vi "PWM Output DAQ Engine.vi"(8 "error in":errorcluster, 10 "DAQ Engine":refnum<notifier>, 11 "Sequence Context In":refnum<k7>) -> (0 "error out":errorcluster)   [LabVIEW 2023, in "LTT_TeststandSteptypes.lvlib"]
uses:
  LTT_TeststandSteptypes.lvlib
  HardwareAbstractionLayer_LVOOP/Main/Class Ref.ctl
  HardwareAbstractionLayer_LVOOP/DMM/DMM.lvclass
  HardwareAbstractionLayer_LVOOP/Function Generator/Function Generator.lvclass
  HardwareAbstractionLayer_LVOOP/Oscilloscope/Oscilloscope.lvclass
  HardwareAbstractionLayer_LVOOP/PowerSupply/PowerSupply.lvclass
  HardwareAbstractionLayer_LVOOP/Teststand/Teststand.lvclass
  HardwareAbstractionLayer_LVOOP/Analog Output/AO/AO.lvclass
  HardwareAbstractionLayer_LVOOP/Analog Input/AI/AI.lvclass
  HardwareAbstractionLayer_LVOOP/Database/Database.lvclass
  HardwareAbstractionLayer_LVOOP/Digital Output/DO_class/DO.lvclass
  HardwareAbstractionLayer_LVOOP/Digital Input/DI_class/DI.lvclass
  HardwareAbstractionLayer_LVOOP/PWM Output/PWM Output_class/PWM Output.lvclass
  HardwareAbstractionLayer_LVOOP/PWM Input/PWM Input_class/PWM Input.lvclass
  HardwareAbstractionLayer_LVOOP/NI Switch/NISwitch_class/NISwitch.lvclass
  HardwareAbstractionLayer_LVOOP/Modbus/Modbus_class/Modbus.lvclass
  HardwareAbstractionLayer_LVOOP/CAN/CAN Lib/CAN_class/CAN.lvclass
  HardwareAbstractionLayer_LVOOP/PWM Output/NI PWM Output_class/NI PWM Output.lvclass
  D:/eDCU LTT/VT LTT Project/Source Code/HardwareAbstractionLayer_LVOOP/PWM Output/PWM Output_class/PWM Output.lvclass
  HardwareAbstractionLayer_LVOOP/Main/Class Options.ctl
  PWM Output/Control/PWM Output Data.ctl
  <vilib>/Utility/error.llb/DialogType.ctl
  HardwareAbstractionLayer_LVOOP/Main/Main.lvclass
  D:/eDCU LTT/VT LTT Project/Source Code/HardwareAbstractionLayer_LVOOP/PWM Output/NI PWM Output_class/NI PWM Output.lvclass
panel:
  in  "stop":bool
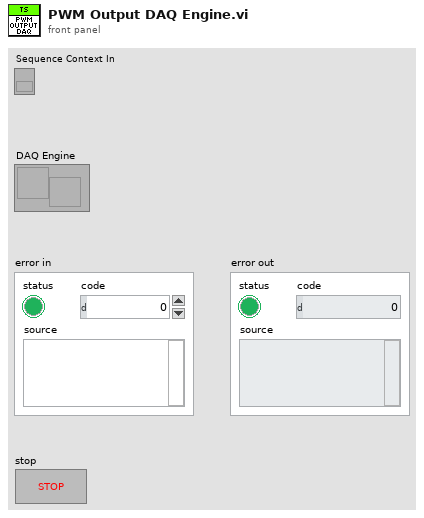
[diagram p1: front panel]
types:
  T1 = typedef "HardwareAbstractionLayer_LVOOP.lvlib/Main.lvclass/Class Ref.ctl" = cluster{"DMM":refnum<class "DMM.lvclass">, "Function Generator":refnum<class "Function Generator.lvclass">, "Oscilloscope":refnum<class "Oscilloscope.lvclass">, "PowerSupply":refnum<class "PowerSupply.lvclass">, "Teststand":refnum<class "Teststand.lvclass">, "AO":refnum<class "AO.lvclass">, "AI":refnum<class "AI.lvclass">, "Database":refnum<class "Database.lvclass">, "AO Waveform Generation":refnum<class "AO.lvclass">, "DO":refnum<class "DO.lvclass">, "DI":refnum<class "DI.lvclass">, "PWM Output":refnum<class "PWM Output.lvclass">, "PWM Input":refnum<class "PWM Input.lvclass">, "RelayOutput":refnum<class "NISwitch.lvclass">, "Modbus":refnum<class "Modbus.lvclass">, "CAN":refnum<class "CAN.lvclass">}
  T2 = typedef "HardwareAbstractionLayer_LVOOP.lvlib/Main.lvclass/Class Options.ctl" = enum16{"Init All Class", "Read All Class", "Write AI Class", "Write AO Class", "Write AO Waveform Generation", "Write DI Class", "Write DO Class", "Write PWM Input Class", "Write PWM Output Class", "Exit"}
  T3 = typedef "LTT_TeststandSteptypes.lvlib/PWM Output Data.ctl" = cluster{"Frequency":dbl, "Duty Cycle":dbl, "PWM Action":enum16{"PWM Start", "PWM Stop"}}
  T4 = typedef "DialogType.ctl" = u16
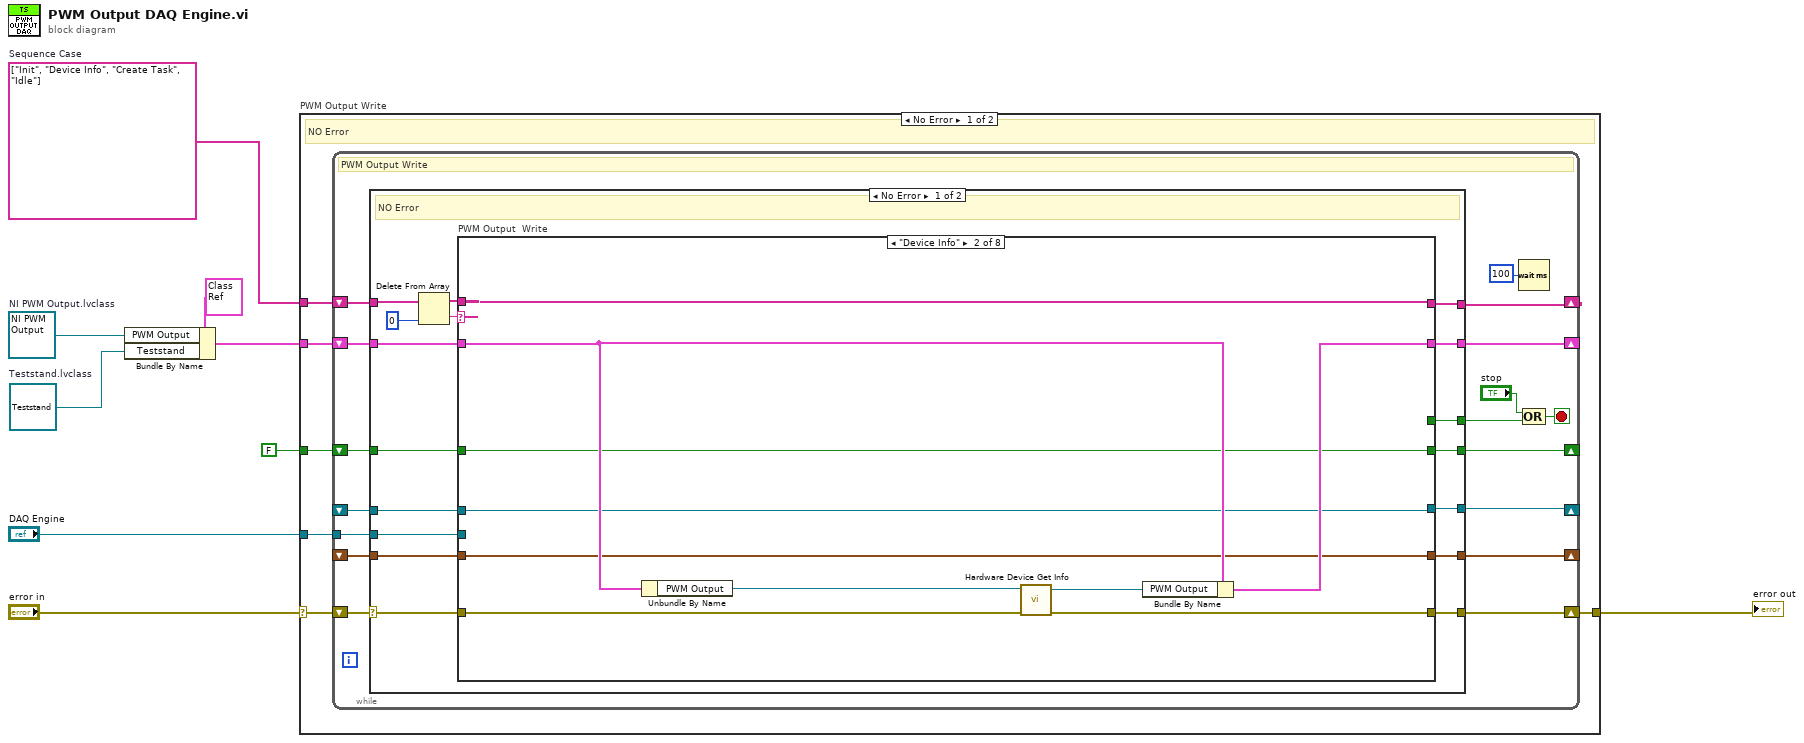
[diagram p0: block diagram]
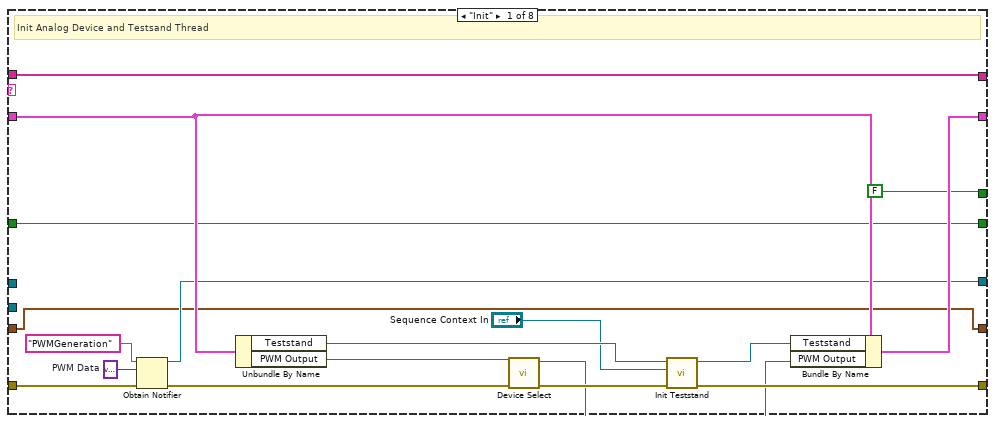
[diagram p2: hidden frame]
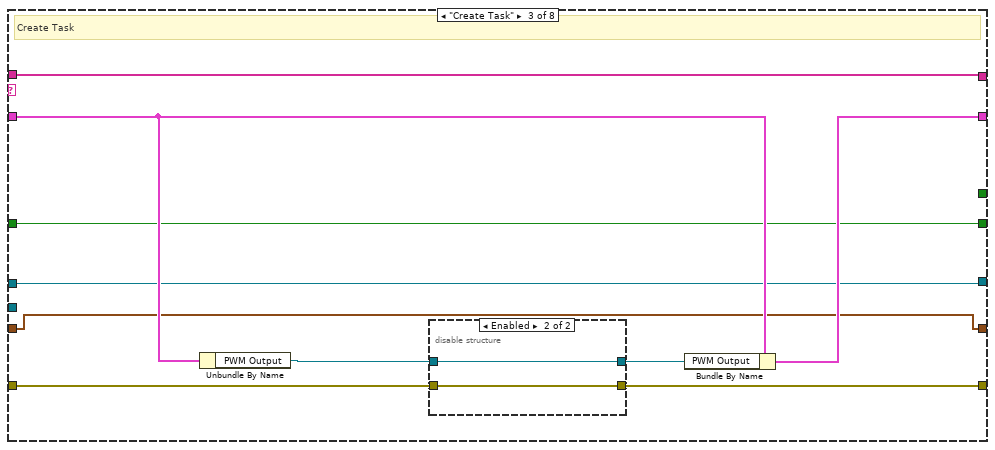
[diagram p3: hidden frame]
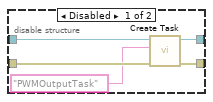
[diagram p4: hidden frame]
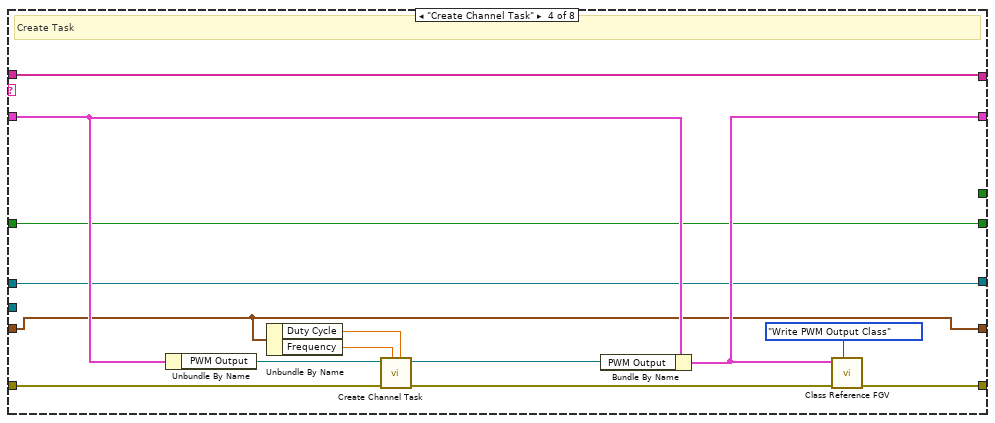
[diagram p5: hidden frame]
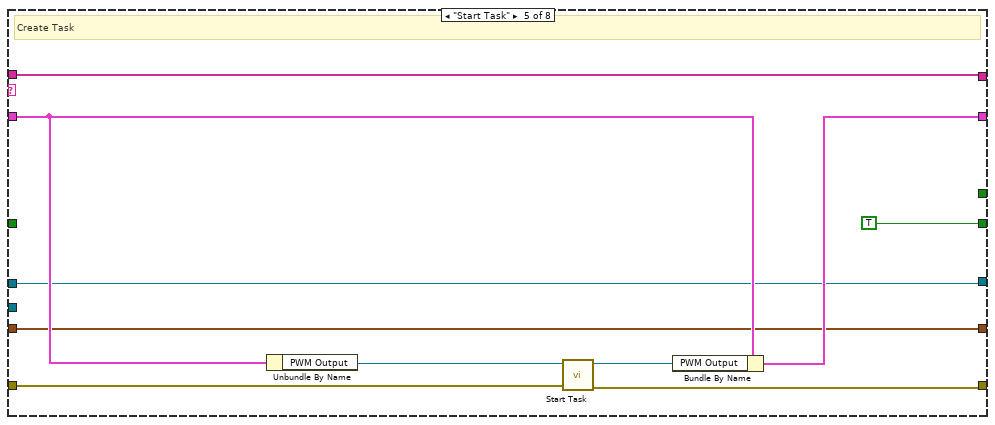
[diagram p6: hidden frame]
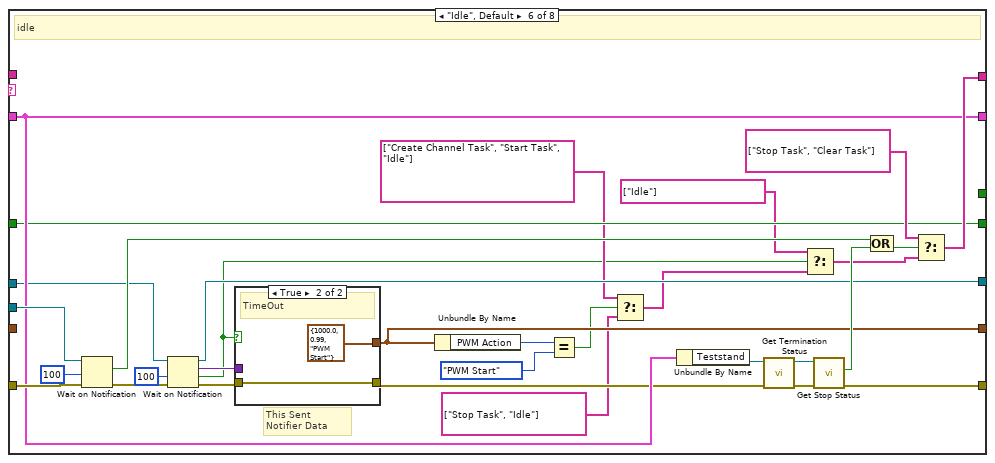
[diagram p7: hidden frame]
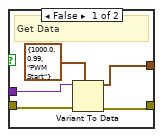
[diagram p8: hidden frame]
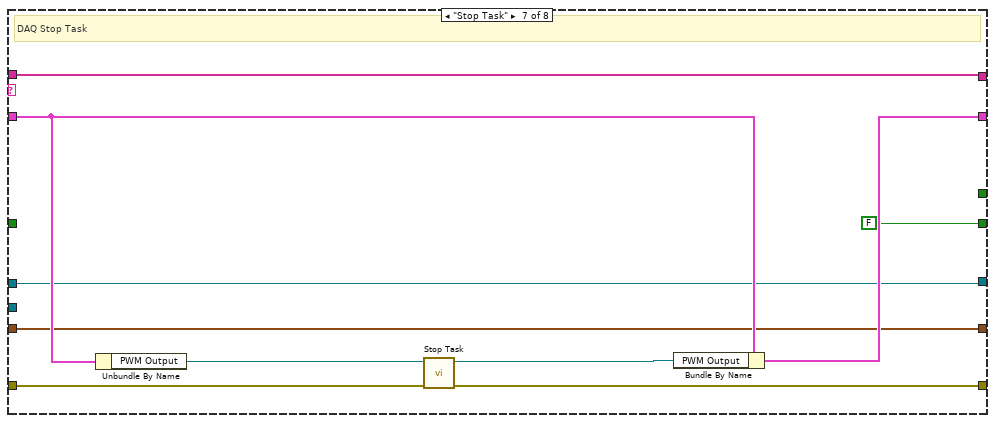
[diagram p9: hidden frame]
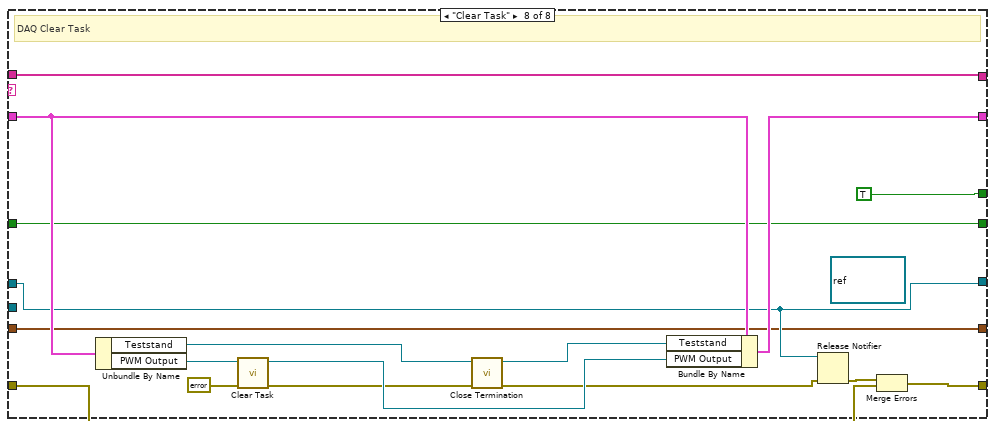
[diagram p10: hidden frame]
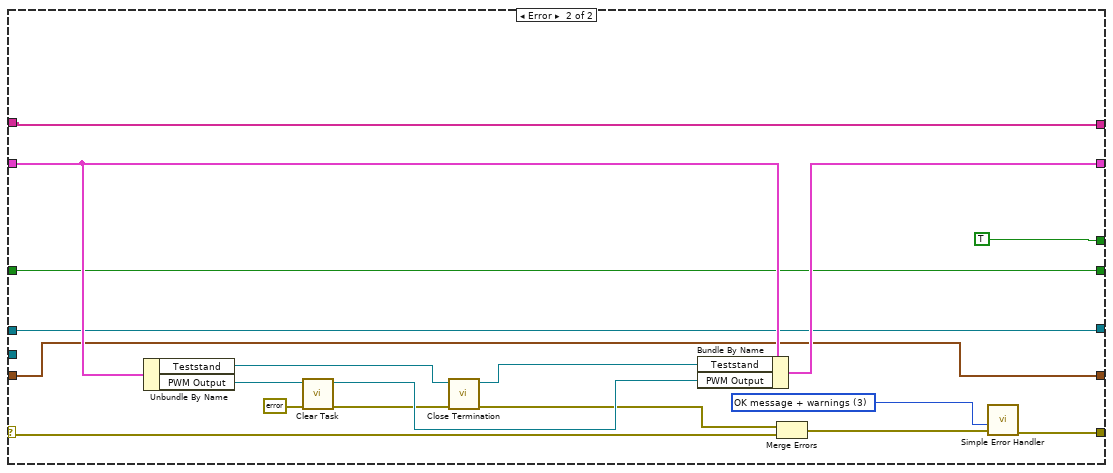
[diagram p11: hidden frame]
diagram:
  w4 = refnum<class "Teststand.lvclass"> refnum  # Teststand.lvclass
  w5 = refnum<class "NI PWM Output.lvclass"> refnum  # NI PWM Output.lvclass
  w7 = string[] ["Init", "Device Info", "Create Task", "Idle"]  # Sequence Case
  n1 = Bundle By Name(cluster=T1 {"DMM"=refnum, "Function Generator"=refnum, "Oscilloscope"=refnum, "PowerSupply"=refnum, "Teststand"=refnum, "AO"=refnum, "AI"=refnum, "Database"=refnum, "AO Waveform Generation"=refnum, "DO"=refnum, "DI"=refnum, "PWM Output"=refnum, "PWM Input"=refnum, "RelayOutput"=refnum, "Modbus"=refnum, "CAN"=refnum} ("Class Cluster"), "PWM Output"=w5, "Teststand"=w4) -> (w8:T1)
  n2 = case "PWM Output Write" shown="No Error" "error in" {
    selector: "error in" -> [w15 w202]
    tunnel: [w14 w202] -> w1
    tunnel: w8 -> [w13 _]
    tunnel: w7 -> [w12 _]
    tunnel: "DAQ Engine" -> [w11 _]
    tunnel: FALSE -> [w10 _]
    frame No Error {
      # "NO Error"
      n3 = while {
        shift-right: [w31] -> w14
        shift-left: w15 -> [w32]
        shift-right: [w29] -> _
        shift-left: w13 -> [w30]
        shift-right: [w27] -> _
        shift-left: w12 -> [w28]
        tunnel: w11 -> [w22]
        shift-right: [w21] -> _
        shift-left: _ -> [w20]
        shift-right: [w18] -> _
        shift-left: w10 -> [w19]
        shift-right: [w17] -> _
        shift-left: _ -> [w16]
        stop <- w24 stop-if-true
        # "PWM Output Write"
        n4 = case shown="No Error" w32 {
          selector: w32 -> [w49 w193]
          tunnel: [w48 w187] -> w31
          tunnel: w30 -> [w44 w191]
          tunnel: [w43 w192] -> w29
          tunnel: w28 -> [w47 w190]
          tunnel: [w41 w190] -> w27
          tunnel: [w40 TRUE] -> w23
          tunnel: w22 -> [w39 _]
          tunnel: [w38 w189] -> w21
          tunnel: w20 -> [w37 w189]
          tunnel: w19 -> [w36 w185]
          tunnel: [w35 w185] -> w18
          tunnel: [w34 w184] -> w17
          tunnel: w16 -> [w33 w184]
          frame No Error {
            # "NO Error"
            n5 = Delete From Array(array=w47, index=0) -> (deleted portion=w46:string, array with subset deleted=w42:string[])  [unwired: 1 in]
            n6 = case "PWM Output  Write" shown="\"Device Info\"" w46 {
              tunnel: w49 -> [w55 w74 w84 w106 w115 w149 w163 w172]
              tunnel: [w59 w73 w83 w102 w113 w142 w158 w173] -> w48
              tunnel: w44 -> [w66 w76 w86 w107 w117 w140 w165 w182]
              tunnel: [w65 w75 w85 w100 w116 w140 w164 w181] -> w43
              tunnel: w42 -> [w67 w77 w87 w108 w118 _ w166 w183]
              tunnel: [w67 w77 w87 w108 w118 w147 w166 w183] -> w41
              tunnel: [FALSE _ _ _ _ _ _ TRUE] -> w40
              tunnel: w39 -> [_ _ _ _ _ w145 _ _]
              tunnel: [w53 w70 w80 w99 w111 w136 w161 w171] -> w38
              tunnel: w37 -> [_ w70 w80 w99 w111 w130 w161 w171]
              tunnel: w36 -> [w52 w69 w79 w98 _ w134 _ w168]
              tunnel: [w52 w69 w79 w98 TRUE w134 FALSE w168] -> w35
              tunnel: [w50 w68 w78 w97 w109 w129 w157 w167] -> w34
              tunnel: w33 -> [w50 w68 w78 w97 w109 _ w157 w167]
              frame "Init" {
                w51 = variant  # PWM Data
                # "Init Analog Device and Testsand Thread"
                n7 = Obtain Notifier(name (unnamed)="PWMGeneration", notification data type=w51, error in (no error)=w55) -> (notifier out=w53:refnum<notifier>, error out=w54:errorcluster)  [unwired: 1 in, 1 out]
                n8 = Unbundle By Name(w66) -> ("Teststand"=w62:refnum<class "Teststand.lvclass">, "PWM Output"=w63:refnum<class "PWM Output.lvclass">)
                n9 = call-dynamic "Device Select.vi"("error in (no error)"=w54, "PWM Output in"=w63) -> ("error out"=w60:errorcluster, "PWM Output out"=w57:refnum<class "PWM Output.lvclass">)  [unwired: 8 in]
                n10 = call-dynamic "Init Teststand.vi"("error in (no error)"=w60, "Sequence Context In"="Sequence Context In", "Teststand in"=w62) -> ("error out"=w59:errorcluster, "Teststand out"=w58:refnum<class "Teststand.lvclass">)  [unwired: 7 in]
                n11 = Bundle By Name(cluster=w66, "Teststand"=w58, "PWM Output"=w57) -> (w65:T1)
              }
              frame "Device Info" {
                n12 = Unbundle By Name(w76) -> ("PWM Output"=w71:refnum<class "PWM Output.lvclass">)
                n13 = call-dynamic "Hardware Device Get Info.vi"("error in (no error)"=w74, "PWM Output in"=w71) -> ("error out"=w73:errorcluster, "PWM Output out"=w72:refnum<class "PWM Output.lvclass">)  [unwired: 8 in]
                n14 = Bundle By Name(cluster=w76, "PWM Output"=w72) -> (w75:T1)
              }
              frame "Create Task" {
                # "Create Task"
                n15 = Unbundle By Name(w86) -> ("PWM Output"=w81:refnum<class "PWM Output.lvclass">)
                n16 = disable-structure shown="Enabled" {
                  disable-tunnel: w84 -> [w92 w93]
                  disable-tunnel: [w91 w93] -> w83
                  disable-tunnel: [w90 w94] -> w82
                  disable-tunnel: w81 -> [w89 w94]
                  frame Disabled {
                    n17 = call-dynamic "Create Task.vi"("error in (no error)"=w92, "Task name"="PWMOutputTask", "PWM Output in"=w89) -> ("error out"=w91:errorcluster, "PWM Output out"=w90:refnum<class "PWM Output.lvclass">)  [unwired: 7 in]
                  }
                  frame Enabled {
                  }
                }
                n18 = Bundle By Name(cluster=w86, "PWM Output"=w82) -> (w85:T1)
              }
              frame "Create Channel Task" {
                # "Create Task"
                n19 = Unbundle By Name(w107) -> ("PWM Output"=w104:refnum<class "PWM Output.lvclass">)
                n20 = Unbundle By Name(w97) -> ("Duty Cycle"=w95:dbl, "Frequency"=w96:dbl)
                n21 = call-dynamic "Create Channel Task.vi"("Duty cycle"=w95, "Frequency"=w96, "error in (no error)"=w106, "PWM Output in"=w104) -> ("error out"=w103:errorcluster, "PWM Output out"=w105:refnum<class "PWM Output.lvclass">)  [unwired: 6 in]
                n22 = Bundle By Name(cluster=w107, "PWM Output"=w105) -> (w100:T1)
                n23 = call "Class Reference FGV.vi"("Options"=Class_Options."Write PWM Output Class", "error in"=w103, "Class Cluster In"=w100) -> ("error out"=w102:errorcluster)  [unwired: 7 in, 1 out]
              }
              frame "Start Task" {
                # "Create Task"
                n24 = Unbundle By Name(w117) -> ("PWM Output"=w114:refnum<class "PWM Output.lvclass">)
                n25 = call-dynamic "Start Task.vi"("error in (no error)"=w115, "PWM Output in"=w114) -> ("error out"=w113:errorcluster, "PWM Output out"=w112:refnum<class "PWM Output.lvclass">)  [unwired: 8 in]
                n26 = Bundle By Name(cluster=w117, "PWM Output"=w112) -> (w116:T1)
              }
              frame "Idle", Default {
                # "This Sent Notifier Data"
                # "idle"
                n27 = Wait on Notification(notifier=w145, timeout in ms (-1)=100, error in (no error)=w149) -> (notification=w144:bool, error out=w137:errorcluster)  [unwired: 1 in, 2 out]
                n28 = Wait on Notification(notifier=w130, timeout in ms (-1)=100, error in (no error)=w137) -> (notifier out=w136:refnum<notifier>, notification=w138:variant, timed out?=w119:bool, error out=w139:errorcluster)  [unwired: 1 in]
                n29 = case shown="True" w119 {
                  tunnel: w139 -> [w154 w156]
                  tunnel: w138 -> [w153 _]
                  tunnel: [w152 w156] -> w135
                  tunnel: [w151 T3 {"Frequency"=1000.0, "Duty Cycle"=0.99, "PWM Action"=enum."PWM Start"} ("PWM Data")] -> w129
                  frame False {
                    # "Get Data"
                    n30 = Variant To Data(error in=w154, type=T3 {"Frequency"=1000.0, "Duty Cycle"=0.99, "PWM Action"=enum."PWM Start"} ("PWM Data"), Variant=w153) -> (data=w151:T3, error out=w152:errorcluster)
                  }
                  frame True {
                    # "TimeOut"
                  }
                }
                n31 = Unbundle By Name(w129) -> ("PWM Action"=w128:enum16{"PWM Start", "PWM Stop"})
                n32 = Equal?(x=w128, y=enum16{"PWM Start", "PWM Stop"}."PWM Start") -> (x = y?=w126:bool)
                n33 = Select(t=string[] ["Create Channel Task", "Start Task", "Idle"], s=w126, f=string[] ["Stop Task", "Idle"]) -> (s? t:f=w121:string[])
                n34 = Unbundle By Name(w140) -> ("Teststand"=w143:refnum<class "Teststand.lvclass">)
                n35 = call-dynamic "Get Termination Status.vi"("error in (no error)"=w135, "Teststand in"=w143) -> ("error out"=w132:errorcluster, "Teststand out"=w133:refnum<class "Teststand.lvclass">)  [unwired: 7 in, 1 out]
                n36 = Select(t=string[] ["Idle"], s=w119, f=w121) -> (s? t:f=w122:string[])
                n37 = call-dynamic "Get Stop Status.vi"("error in (no error)"=w132, "Teststand in"=w133) -> ("error out"=w142:errorcluster, "Value"=w141:bool)  [unwired: 7 in, 1 out]
                n38 = Compound Arithmetic op=OR(w144, w141) -> (w146:bool)
                n39 = Select(t=string[] ["Stop Task", "Clear Task"], s=w146, f=w122) -> (s? t:f=w147:string[])
              }
              frame "Stop Task" {
                # "DAQ Stop Task"
                n40 = Unbundle By Name(w165) -> ("PWM Output"=w162:refnum<class "PWM Output.lvclass">)
                n41 = call-dynamic "Stop Task.vi"("error in (no error)"=w163, "PWM Output in"=w162) -> ("error out"=w158:errorcluster, "PWM Output out"=w159:refnum<class "PWM Output.lvclass">)  [unwired: 8 in]
                n42 = Bundle By Name(cluster=w165, "PWM Output"=w159) -> (w164:T1)
              }
              frame "Clear Task" {
                (unwired) refnum<notifier> refnum ("notifier out")
                # "DAQ Clear Task"
                n43 = Unbundle By Name(w182) -> ("Teststand"=w177:refnum<class "Teststand.lvclass">, "PWM Output"=w179:refnum<class "PWM Output.lvclass">)
                n44 = call-dynamic "Clear Task.vi"("error in (no error)"=errorcluster {"status"=FALSE, "code"=0, "source"=""}, "PWM Output in"=w179) -> ("error out"=w176:errorcluster, "PWM Output out"=w178:refnum<class "PWM Output.lvclass">)  [unwired: 8 in]
                n45 = call-dynamic "Close Termination.vi"("error in (no error)"=w176, "Teststand in"=w177) -> ("error out"=w170:errorcluster, "Teststand out"=w175:refnum<class "Teststand.lvclass">)  [unwired: 8 in]
                n46 = Bundle By Name(cluster=w182, "Teststand"=w175, "PWM Output"=w178) -> (w181:T1)
                n47 = Release Notifier(notifier=w171, error in (no error)=w170) -> (error out=w169:errorcluster)  [unwired: 1 in, 2 out]
                n48 = Merge Errors(w169, w172) -> (w173:errorcluster)
              }
            }
          }
          frame Error {
            w186 = T4 3 items=["no dialog", "OK message", "continue or stop message", "OK message + warnings", "continue/stop + warnings"] ("type of dialog (OK msg:1)")
            n49 = Unbundle By Name(w191) -> ("Teststand"=w198:refnum<class "Teststand.lvclass">, "PWM Output"=w200:refnum<class "PWM Output.lvclass">)
            n50 = call-dynamic "Clear Task.vi"("error in (no error)"=errorcluster {"status"=FALSE, "code"=0, "source"=""}, "PWM Output in"=w200) -> ("error out"=w197:errorcluster, "PWM Output out"=w199:refnum<class "PWM Output.lvclass">)  [unwired: 8 in]
            n51 = call-dynamic "Close Termination.vi"("error in (no error)"=w197, "Teststand in"=w198) -> ("error out"=w195:errorcluster, "Teststand out"=w196:refnum<class "Teststand.lvclass">)  [unwired: 8 in]
            n52 = Bundle By Name(cluster=w191, "Teststand"=w196, "PWM Output"=w199) -> (w192:T1)
            n53 = Merge Errors(w195, w193) -> (w188:errorcluster)
            n54 = call <vilib>:"Simple Error Handler.vi"("type of dialog (OK msg:1)"=w186, "error in (no error)"=w188) -> ("error out"=w187:errorcluster)  [unwired: 3 in, 4 out]
          }
        }
        n55 = Wait (ms)(milliseconds to wait=u32 100) -> ()  [unwired: 1 out]
        n56 = Compound Arithmetic op=OR("stop", w23) -> (w24:bool)
      }
    }
    frame Error {
      # "Error"
    }
  }
  "error out" <- w1
